vi "lookupImage.vi"(8 "error in (no error)":errorcluster, 11 "ImageStreamViewer in":refnum<class "ImageStreamViewer.lvclass">) -> (0 "error out":errorcluster, 3 "ImageStreamViewer out":refnum<class "ImageStreamViewer.lvclass">)   [LabVIEW 2011, in "Views.lvlib" / "Camera.lvlib" / "ImageStreamViewer.lvclass"]
uses:
  ImageStreamViewer.lvclass
  ImageStreamViewer.lvclass/ImageStreamViewer.ctl
panel:
  # "The user wants to look at a different image.\naccess the image path for the scroll position,\nand update the displays"
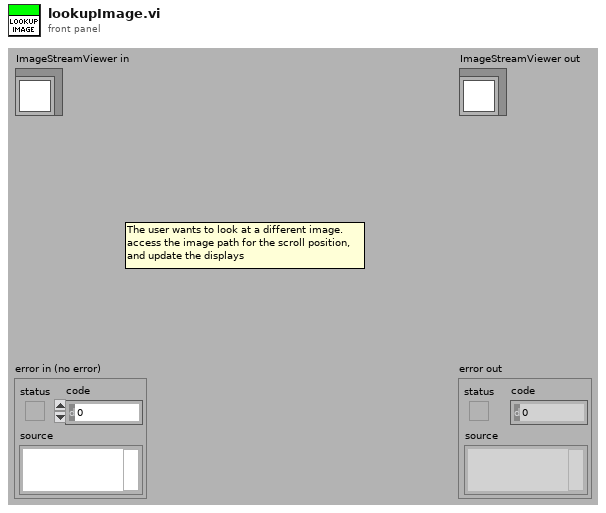
[diagram p1: front panel]
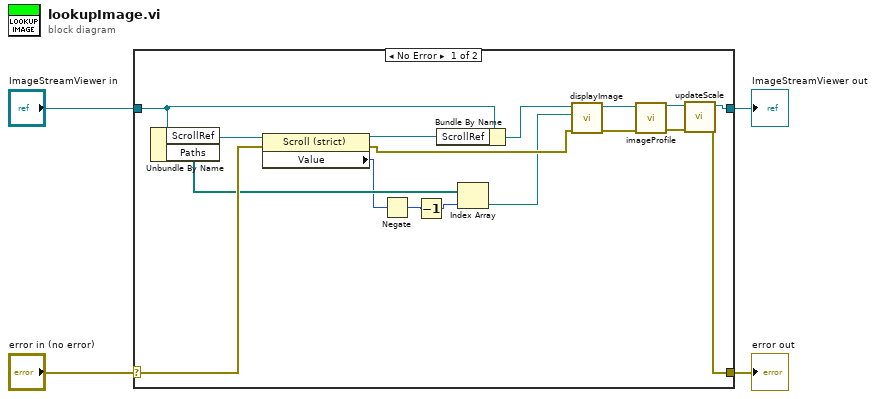
[diagram p0: block diagram]
diagram:
  n1 = case shown="No Error" "error in (no error)" {
    selector: "error in (no error)" -> [w20 w23]
    tunnel: [w7 w23] -> w3
    tunnel: [w5 w22] -> w1
    tunnel: "ImageStreamViewer in" -> [w14 w22]
    frame No Error {
      n2 = Unbundle By Name(w14) -> ("ScrollRef"=w21:refnum<vi>, "Paths"=w19:path[])
      n3 = property class="Scroll (strict)"(reference=w21, error in=w20) -> (reference out=w15:refnum<vi>, error out=w12:errorcluster, "Value"=w16:i32)
      n4 = Negate(x=w16) -> (-x=w18:i32)
      n5 = Decrement(x=w18) -> (x-1=w17:i32)
      n6 = Bundle By Name(cluster=w14, "ScrollRef"=w15) -> (w13:refnum<class "ImageStreamViewer.lvclass">)
      n7 = Index Array(array=w19, index=w17) -> (element=w11:path)
      n8 = call "displayImage.vi"("error in (no error)"=w12, "Path"=w11, "ImageStreamViewer in"=w13) -> ("error out"=w9:errorcluster, "ImageStreamViewer out"=w10:refnum<class "ImageStreamViewer.lvclass">)  [unwired: 7 in]
      n9 = call "imageProfile.vi"("error in (no error)"=w9, "ImageStreamViewer in"=w10) -> ("error out"=w8:errorcluster, "ImageStreamViewer out"=w6:refnum<class "ImageStreamViewer.lvclass">)  [unwired: 8 in]
      n10 = call "updateScale.vi"("error in (no error)"=w8, "ImageStreamViewer in"=w6) -> ("error out"=w7:errorcluster, "ImageStreamViewer out"=w5:refnum<class "ImageStreamViewer.lvclass">)  [unwired: 8 in]
    }
    frame Error {
    }
  }
  "error out" <- w3
  "ImageStreamViewer out" <- w1
